vi "E11_Srings.vi"() -> ()   [LabVIEW 2026]
panel:
  out "resulting string":string
  out "offset past match":i32
  out "after substring":string
  out "match substring":string
  out "before substring":string
  out "result string 2":string
  out "result string":string
  out "substring":string
  out "concatenated string":string
  out "length":i32
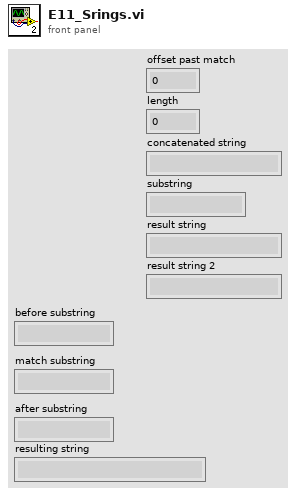
[diagram p1: front panel]
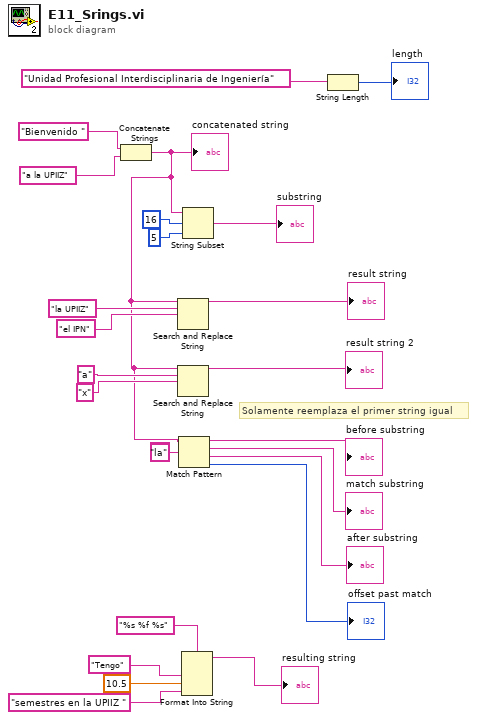
[diagram p0: block diagram]
diagram:
  (unwired) "la" ("regular expression")
  # "Solamente reemplaza el primer string igual"
  n1 = Concatenate Strings "Concatenate Strings"("Bienvenido ", "a la UPIIZ") -> (w11:string)
  "concatenated string" <- w11
  n2 = Search and Replace String(input string=w11, search string="la UPIIZ", replace string="el IPN") -> (result string=→"result string":string)  [unwired: 5 in, 3 out]
  n3 = Search and Replace String(input string=w11, search string="a", replace string="x") -> (result string=→"result string 2":string)  [unwired: 5 in, 3 out]
  n4 = Match Pattern(string=w11, regular expression="la") -> (before substring=→"before substring":string, match substring=→"match substring":string, after substring=→"after substring":string, offset past match=→"offset past match":i32)  [unwired: 1 in]
  n5 = Format Into String "Format Into String"(format string="%s %f %s", "Tengo" ("regular expression"), 10.5 ("input 2"), "semestres en la UPIIZ " ("regular expression")) -> (resulting string=→"resulting string":string)  [unwired: 2 in, 1 out]
  n6 = String Subset(string=w11, offset (0)=16, length (rest)=5 ("length (rest)")) -> (substring=→"substring":string)
  n7 = String Length(string="Unidad Profesional Interdisciplinaria de Ingeniería") -> (length=→"length":i32)
